vi "Import and Export Controls.vi"() -> ()   [LabVIEW 2013, in "DCAF UI Elements.lvlib"]
uses:
  Controls/DCAF UI Elements.lvlib
  Controls/Export.ctl
  Controls/Import.ctl
panel:
  in  "Import":T1
  in  "Export":T2
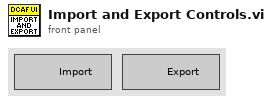
[diagram p1: front panel]
types:
  T1 = typedef "DCAF UI Elements.lvlib/Import.ctl" = bool
  T2 = typedef "DCAF UI Elements.lvlib/Export.ctl" = bool
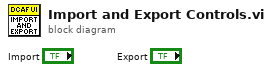
[diagram p0: block diagram]
diagram:
